vi "RandomBytes.vi"(1 "N":i32) -> (0 "N Random Bytes":u8[](array[numeric]) format="%08b")   [LabVIEW 2017, in "GPNumeric.lvlib"]
doc: "Generates <B>N Random Bytes</B>. With this you can create a random bit sequence of any size.\n\nThis VI is inlined.\n\nSteen Schmidt\nGPower\n18/12 2016"
uses:
  GPNumeric.lvlib
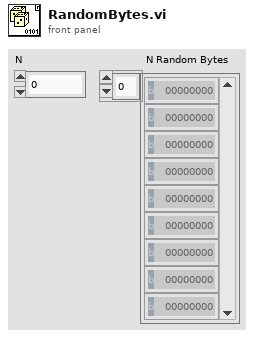
[diagram p1: front panel]
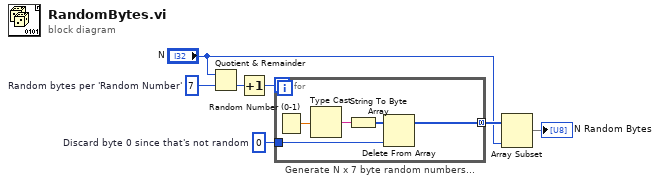
[diagram p0: block diagram]
diagram:
  w5 = 0  # Discard byte 0 since that's not random
  w7 = 7  # Random bytes per 'Random Number'
  n1 = Quotient & Remainder(x="N", y=w7) -> (floor(x/y)=w6:i32)  [unwired: 1 out]
  n2 = Increment(x=w6) -> (x+1=w4:i32)
  n3 = for "Generate N x 7 byte random numbers..." {
    N: w4 -> [_]
    tunnel: w5 -> [w9]
    tunnel: [w8] -> w3 mode=concatenating
    n4 = Random Number (0-1)() -> (number: 0 to 1=w12:dbl)
    n5 = Type Cast(x=w12) -> (*(type *) &x=w11:string)  [unwired: 1 in]
    n6 = String To Byte Array(string=w11) -> (unsigned byte array=w10:u8[])
    n7 = Delete From Array(array=w10, index=w9) -> (array with subset deleted=w8:u8[])  [unwired: 1 in, 1 out]
  }
  n8 = Array Subset(array=w3, length="N") -> (→"N Random Bytes":u8[])  [unwired: 1 in]
